vi "Serial float Read from ATMega32.vi"() -> ()   [LabVIEW 2016]
uses:
  <vilib>/Instr/_visa.llb/VISA Configure Serial Port (Instr).vi
panel:
  in  "Button 8":bool
  in  "Button 7":bool
  in  "Button 6":bool
  in  "Button 5":bool
  in  "Button 4":bool
  in  "Button 3":bool
  in  "Button 2":bool
  in  "Button 1":bool
  out "LED Array":bool[](array[boolean])
  out "Received Value":u8
  out "Sent Value":u8
  out "no of sent bytes":u32
  in  "stop":bool
  in  "COM PORT":refnum<visa-resource-name>
  # "Configuration"
  # "Input From PushButton of ATMega32"
  # "Input to LEDs of ATMega32"
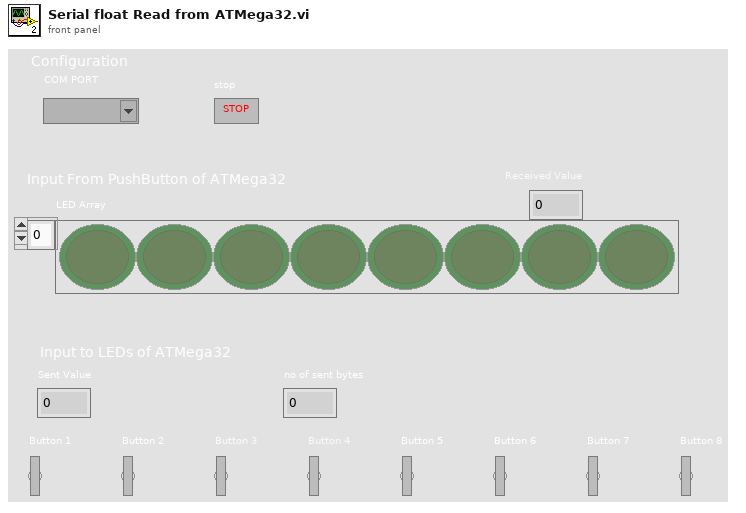
[diagram p1: front panel]
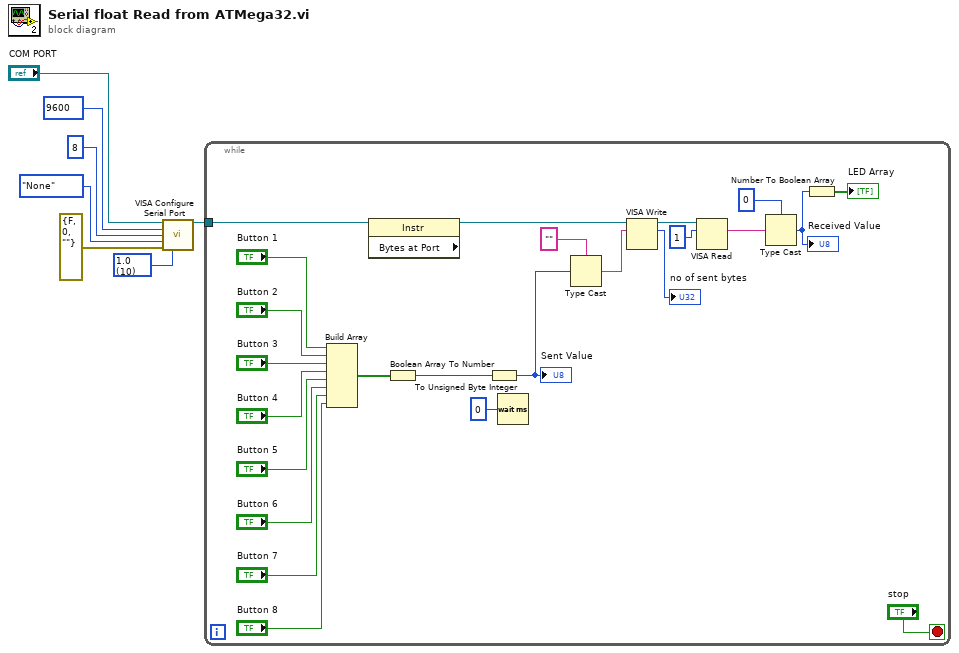
[diagram p0: block diagram]
diagram:
  w2 = u16 10 items=["1.0"=10, "1.5"=15, "2.0"=20] ("stop bits (10: 1 bit)")
  n1 = call-poly "VISA Configure Serial Port"("VISA resource name"="COM PORT", "baud rate (9600)"=u32 9600, "data bits (8)"=u16 8, "parity (0:none)"=enum16{"None", "Odd", "Even", "Mark", "Space"}."None", "error in (no error)"=errorcluster {"status"=FALSE, "code"=0, "source"=""}, "stop bits (10: 1 bit)"=w2) -> ("VISA resource name out"=w1:refnum<visa-resource-name>)  [unwired: 8 in, 1 out]
  n2 = while {
    tunnel: w1 -> [w31]
    stop <- "stop" stop-if-true
    n3 = Build Array("Button 1", "Button 2", "Button 3", "Button 4", "Button 5", "Button 6", "Button 7", "Button 8") -> (w8:bool[])
    n4 = property class="Instr" props=["Bytes at Port"](reference=w31) -> (reference out=w27:refnum<visa-resource-name>)  [unwired: 1 in, 2 out]
    n5 = Boolean Array To Number(Boolean array=w8) -> (number=w26:u32)
    n6 = To Unsigned Byte Integer(number=w26) -> (unsigned 8bit integer=w25:u8)
    "Sent Value" <- w25
    n7 = Wait (ms)(milliseconds to wait=u32 0) -> ()  [unwired: 1 out]
    n8 = Type Cast(type="", x=w25) -> (*(type *) &x=w23:string)
    n9 = VISA Write(VISA resource name=w27, write buffer=w23) -> (VISA resource name out=w18:refnum<visa-resource-name>, return count=→"no of sent bytes":u32)  [unwired: 1 in, 1 out]
    n10 = VISA Read(VISA resource name=w18, byte count=u32 1) -> (read buffer=w21:string)  [unwired: 1 in, 3 out]
    n11 = Type Cast(type=u8 0, x=w21) -> (*(type *) &x=w17:u8)
    "Received Value" <- w17
    n12 = Number To Boolean Array(number=w17) -> (Boolean array=→"LED Array":bool[])
  }
